vi "Save to csv.vi"(8 "error in (no error)":errorcluster, 9 "Array":dbl[][](array[numeric]), 10 "Rate":u16, 11 "file path (dialog if empty)":path) -> (0 "error out":errorcluster)   [LabVIEW 2022 SP3]
uses:
  <vilib>/Utility/file.llb/Write Delimited Spreadsheet (string).vi
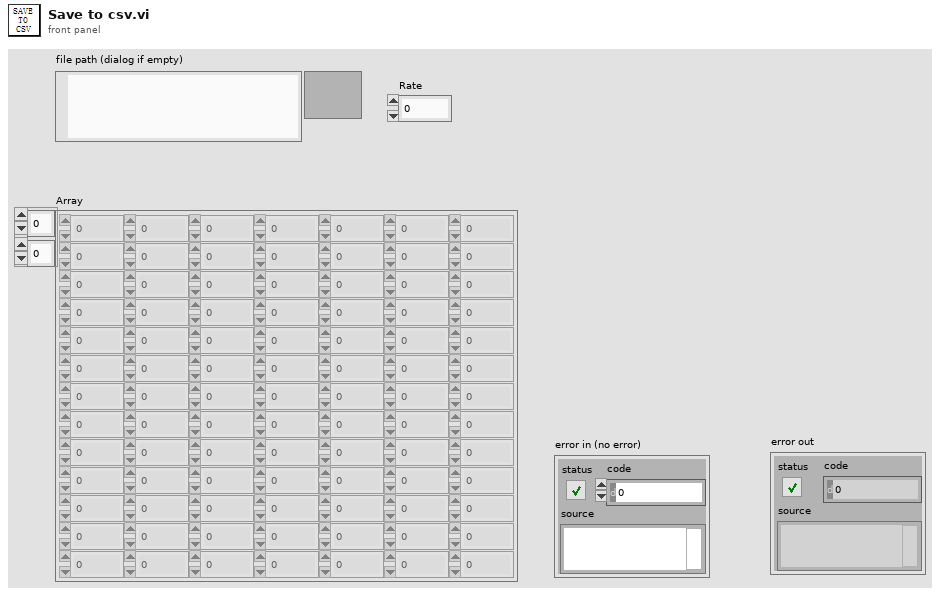
[diagram p1: front panel]
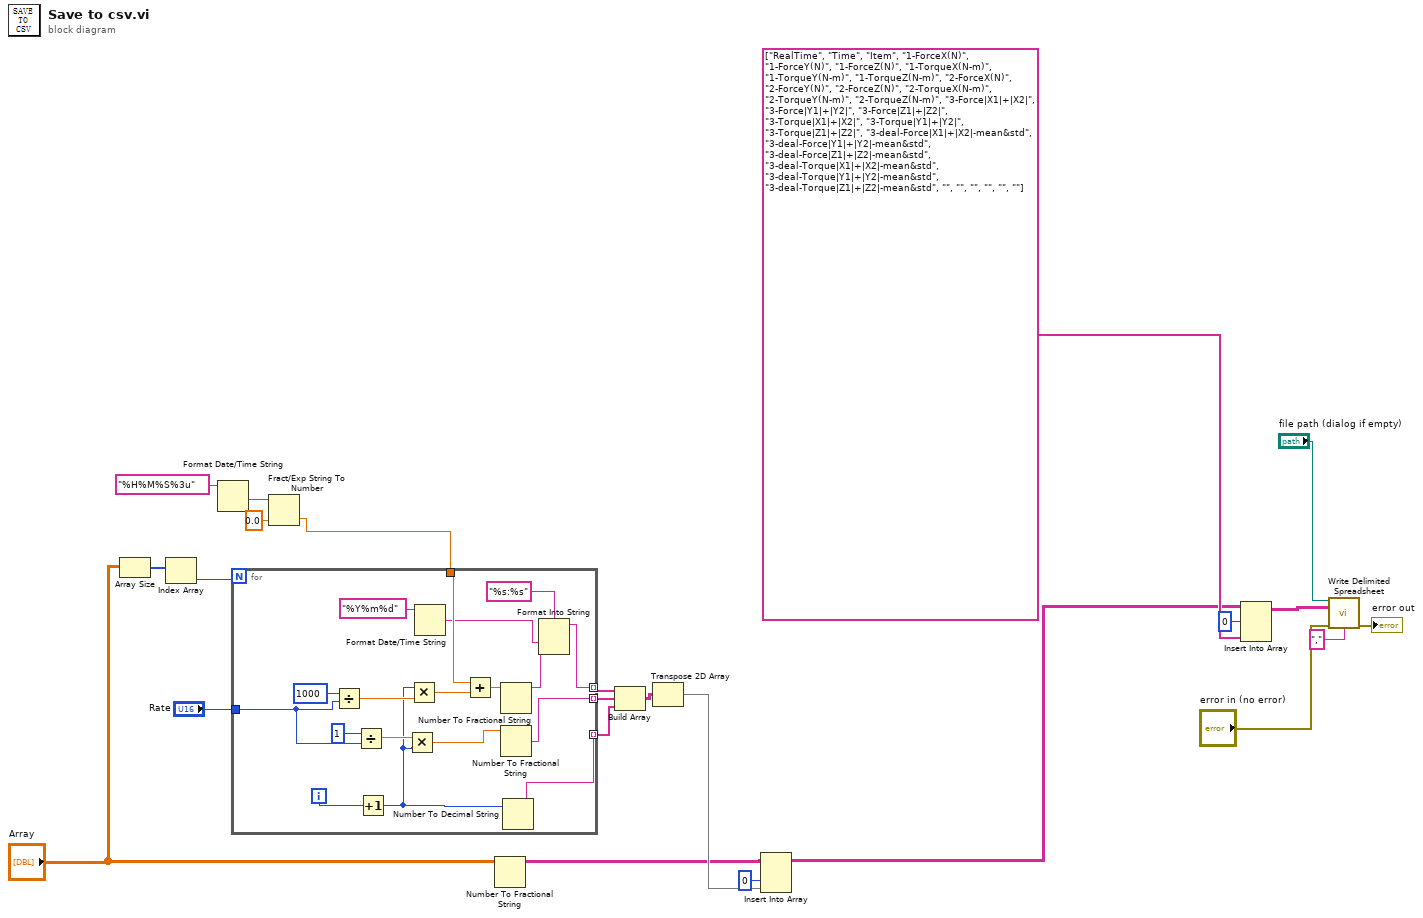
[diagram p0: block diagram]
diagram:
  n1 = Array Size(array="Array") -> (size(s)=w21:i32[])
  n2 = Index Array(array=w21) -> (element=w1:i32)  [unwired: 1 in]
  n3 = Format Date/Time String(time format string (%c)="%H%M%S%3u") -> (date/time string=w22:string)  [unwired: 2 in]
  n4 = Fract/Exp String To Number(string=w22, default (0 dbl)=sgl 0.0 ("default (0 I32)")) -> (number=w20:sgl)  [unwired: 2 in, 1 out]
  n5 = for {
    N: w1 -> [_]
    tunnel: w20 -> [w40]
    tunnel: [w34] -> w17 mode=indexing
    tunnel: [w36] -> w3 mode=indexing
    tunnel: "Rate" -> [w28]
    tunnel: [w30] -> w2 mode=indexing
    i -> [w38]
    n6 = Divide(x=u16 1000, y=w28) -> (x/y=w29:dbl)
    n7 = Divide(x=u16 1, y=w28) -> (x/y=w26:dbl)
    n8 = Increment(x=w38) -> (x+1=w25:i32)
    n9 = Multiply(x=w26, y=w25) -> (x*y=w24:dbl)
    n10 = Multiply(x=w25, y=w29) -> (x*y=w31:dbl)
    n11 = Format Date/Time String(time format string (%c)="%Y%m%d") -> (date/time string=w33:string)  [unwired: 2 in]
    n12 = Add(x=w40, y=w31) -> (x+y=w39:dbl)
    n13 = Number To Fractional String(number=w39) -> (F-format string=w35:string)  [unwired: 3 in]
    n14 = Number To Fractional String(number=w24) -> (F-format string=w30:string)  [unwired: 3 in]
    n15 = Number To Decimal String(number=w25) -> (decimal integer string=w36:string)  [unwired: 1 in]
    n16 = Format Into String(format string="%s:%s", w33, w35) -> (resulting string=w34:string)  [unwired: 2 in, 1 out]
  }
  n17 = Number To Fractional String(number="Array") -> (F-format string=w8:string[][])  [unwired: 3 in]
  n18 = Build Array(w17, w2, w3) -> (w16:string[][])
  n19 = Transpose 2D Array(2D array=w16) -> (transposed array=w11:string[][])
  n20 = Insert Into Array(array=w8, index (col)=0 ("disabled index (col)"), new element=w11) -> (w7:string[][])  [unwired: 1 in]
  n21 = Insert Into Array(array=w7, index (row)=0, new element=string[] ["RealTime", "Time", "Item", "1-ForceX(N)", "1-ForceY(N)", "1-ForceZ(N)", "1-TorqueX(N-m)", "1-TorqueY(N-m)", "1-TorqueZ(N-m)", "2-ForceX(N)", "2-ForceY(N)", "2-ForceZ(N)", "2-TorqueX(N-m)", "2-TorqueY(N-m)", "2-TorqueZ(N-m)", "3-Force|X1|+|X2|", "3-Force|Y1|+|Y2|", "3-Force|Z1|+|Z2|", "3-Torque|X1|+|X2|", "3-Torque|Y1|+|Y2|", "3-Torque|Z1|+|Z2|", "3-deal-Force|X1|+|X2|-mean&std", "3-deal-Force|Y1|+|Y2|-mean&std", "3-deal-Force|Z1|+|Z2|-mean&std", "3-deal-Torque|X1|+|X2|-mean&std", "3-deal-Torque|Y1|+|Y2|-mean&std", "3-deal-Torque|Z1|+|Z2|-mean&std", "", "", "", "", "", ""]) -> (w13:string[][])  [unwired: 1 in]
  n22 = call-poly <vilib>:"Write Delimited Spreadsheet.vi"("file path (dialog if empty)"="file path (dialog if empty)", "2D data"=w13, "error in (no error)"="error in (no error)", "delimiter (\\t)"="," ("delimiter (\\t)")) -> ("error out"=→"error out":errorcluster)  [unwired: 10 in, 1 out]
